vi "日志报警状态存储 (子VI).vi"() -> ()   [LabVIEW 2016, in "斯坦道CODMn.lvlib"]
uses:
  <vilib>/ptbypt/NI_PtbyPt.lvlib
panel:
  out "多列列表框":i32(listbox)
  out "CODMn工作状态":T1(ring)
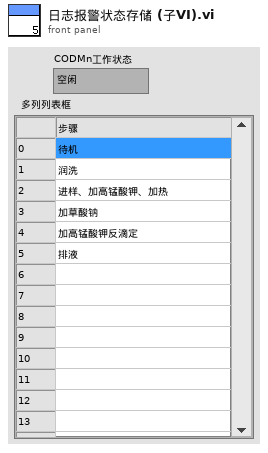
[diagram p1: front panel]
types:
  T1 = enum16{"空闲", "水样测试", "标样核查", "零点核查", "跨度核查", "空白测试", "平行样测试", "质控样", "空白校准", "标样校准", "加标回收"}
  T2 = cluster{"时间标识":timestamp, "设备":string, "日志信息":string, "备注":string}
  T3 = cluster{"时间标识":timestamp, "参数":string, "日志信息":string, "流程参数":string}
  T4 = cluster{"ORP故障":bool, "温控器故障":bool, "加热故障":bool, "高锰酸钾报警":bool, "草酸钠报警":bool, "测量错误":bool, "校零错误":bool, "校标错误":bool, " 进水样超量程":bool, "排液阀故障":bool, "60分钟超时报警":bool, "进样无液体报警":bool}
  T5 = cluster{"时间标识":timestamp, "设备":string, "日志信息":string, "流程参数":string}
  T6 = cluster{"测量量程":dbl, "测量精度":dbl, "测量间隔":dbl, "消解温度":dbl, "消解时长":dbl, "空白校准时间":timestamp, "曲线截距":dbl, "曲线斜率":dbl, "测量检出限":dbl, "测量信号值":dbl, "线性相关系数":dbl, "二次多项式系数":dbl, "标样校准时间":timestamp, "稀释倍数":dbl, "三项式系数":dbl, "空白标定系数":dbl, "量程系数":dbl, "F0/ORPA":dbl, "F1/ORPB":dbl, "F2/ORPK":dbl, "F3":dbl, "F4":dbl, "F5":dbl, "F6":dbl, "F7":dbl, "X0/滴定数":dbl, "量程":dbl}
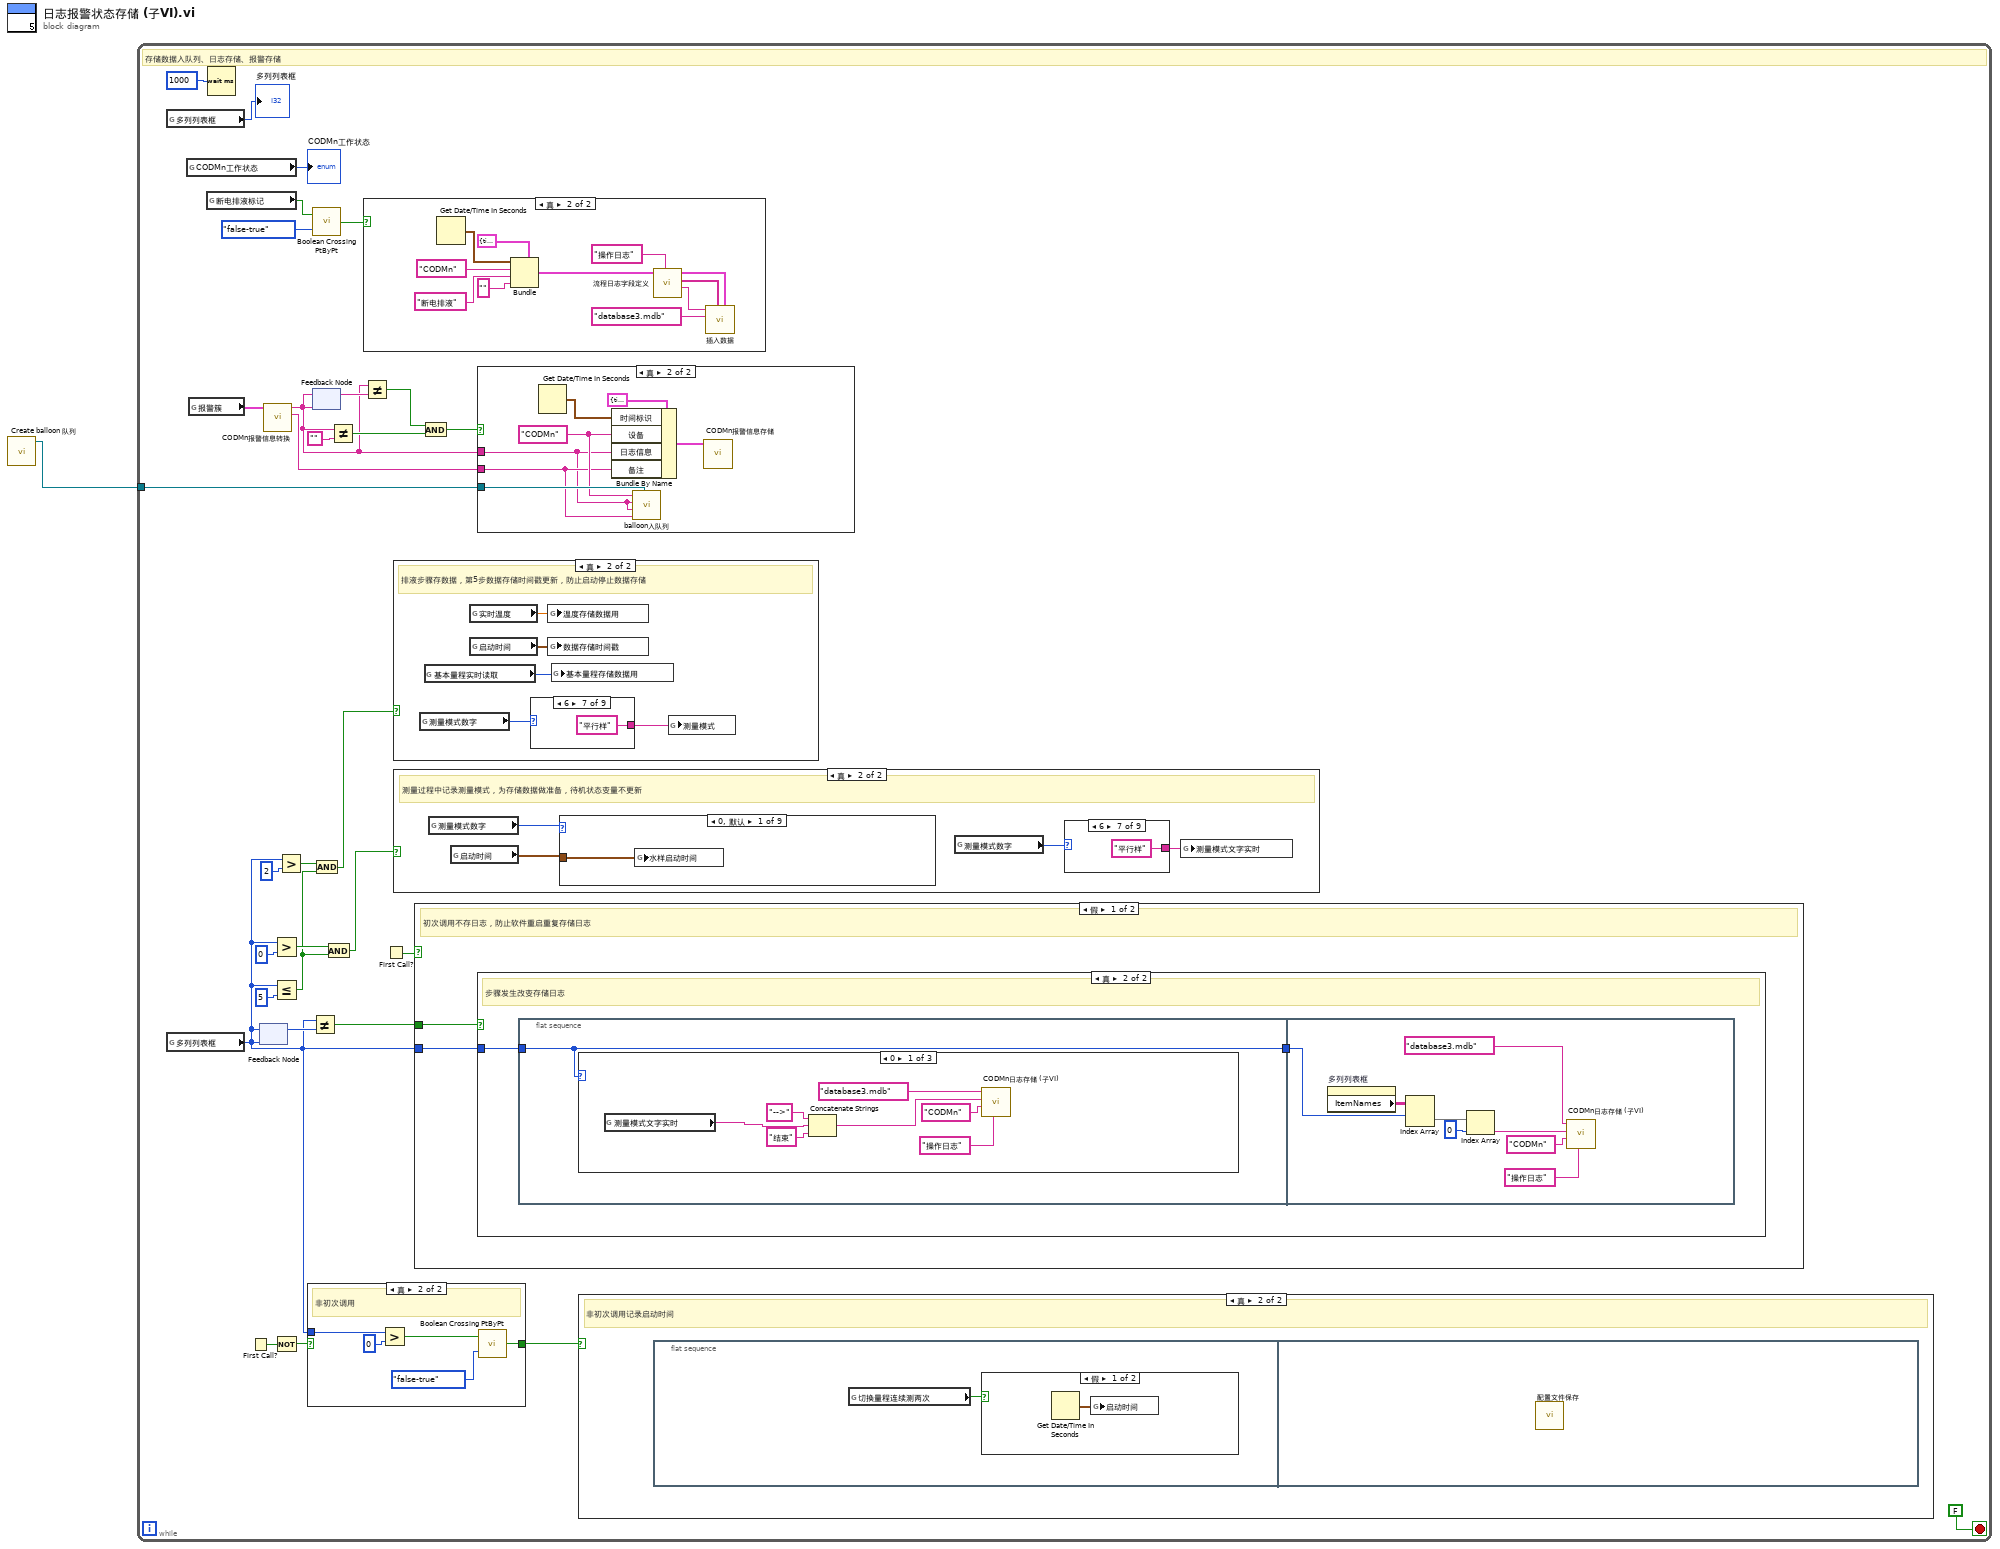
[diagram p0: block diagram]
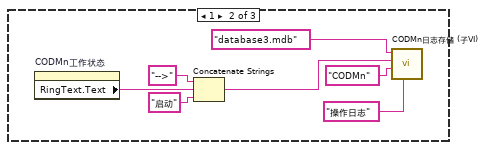
[diagram p3: hidden frame]
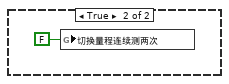
[diagram p10: hidden frame]
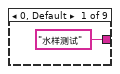
[diagram p12: hidden frame]
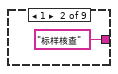
[diagram p13: hidden frame]
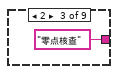
[diagram p14: hidden frame]
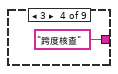
[diagram p15: hidden frame]
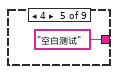
[diagram p16: hidden frame]
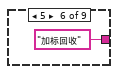
[diagram p17: hidden frame]
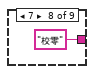
[diagram p18: hidden frame]
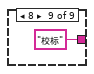
[diagram p19: hidden frame]
diagram:
  n1 = call "Create balloon 队列.vi"() -> ("队列输出"=w1:refnum<queue>)  [unwired: 11 in]
  n2 = while {
    tunnel: w1 -> [w2]
    stop <- FALSE stop-if-true
    # "存储数据入队列、日志存储、报警存储"
    n3 = global read "运行时序全局变量.vi" "多列列表框"() -> (→"多列列表框":i32)
    n4 = global read "运行时序全局变量.vi" "多列列表框"() -> (w6:i32)
    n5 = global read "COD测量模式全局.vi" "CODMn工作状态"() -> (→"CODMn工作状态":T1)
    n6 = global read "COD内部交互全局.vi" "报警簇"() -> (w13:T4)
    n7 = global read "COD内部交互全局.vi" "断电排液标记"() -> (w12:bool)
    n8 = Wait (ms)(milliseconds to wait=u32 1000 ("等待时间（毫秒）")) -> ()  [unwired: 1 out]
    n9 = First Call?() -> (First Call?: T/F=w16:bool)
    n10 = feedback #1(w6) -> (w27:i32)
    n11 = feedback-in #1(w6) -> ()
    n12 = call "CODMn报警信息转换.vi"("报警簇"=w13) -> ("CODMN报警信息备注"=w3:string, "CODMN报警信息"=w17:string)  [unwired: 9 in]
    n13 = Greater?(x=w6, y=u16 0) -> (0:w32:bool)
    n14 = Less Or Equal?(x=w6, y=u16 5) -> (x <= y?=w7:bool)
    n15 = Not(x=w16) -> (.not. x?=w14:bool)
    n16 = Greater?(x=w6, y=u16 2) -> (0:w8:bool)
    n17 = case shown="真" w14 {
      selector: w14 -> [w60 _]
      tunnel: w6 -> [_ w62]
      tunnel: [w60 w61] -> w15
      frame False {
      }
      frame True {
        # "非初次调用"
        n18 = Greater?(x=w62, y=u16 0) -> (0:w65:bool)
        n19 = call <vilib>:"Boolean Crossing PtByPt.vi"("direction"=enum16{"either", "false-true", "true-false"}."false-true", "input"=w65) -> ("crossing"=w61:bool)  [unwired: 1 in]
      }
    }
    n20 = Not Equal?(x=w6, y=w27) -> (x != y?=w28:bool)
    n21 = call <vilib>:"Boolean Crossing PtByPt.vi"("direction"=enum16{"either", "false-true", "true-false"}."false-true", "input"=w12) -> ("crossing"=w23:bool)  [unwired: 1 in]
    n22 = feedback #2(w17) -> (w18:string)
    n23 = feedback-in #2(w17) -> ()
    n24 = And(x=w8, y=w7) -> (x .and. y?=w5:bool)
    n25 = And(x=w32, y=w7) -> (x .and. y?=w4:bool)
    n26 = Not Equal?(x=w17, y="") -> (x != y?=w22:bool)
    n27 = Not Equal?(x=w17, y=w18) -> (x != y?=w19:bool)
    n28 = case shown="真" w23 {
      frame False {
      }
      frame True {
        n29 = Get Date/Time In Seconds() -> (seconds since 1Jan1904=w78:timestamp)
        n30 = Bundle(cluster=T3 {"时间标识"=timestamp(0 s since 1904-01-01), "参数"="", "日志信息"="", "流程参数"=""} ("data in"), "时间标识"=w78, "参数"="CODMn" ("table输入"), "日志信息"="断电排液", "流程参数"="" ("table输入")) -> (w76:T3)
        n31 = call "流程日志字段定义.vi"("table输入"="操作日志", "data in"=w76) -> ("table输出"=w81:string, "columns"=w82:string[], "data out"=w83:T5)  [unwired: 7 in]
        n32 = call "插入数据.vi"("data"=w83, "columns"=w82, "database"="database3.mdb", "table"=w81) -> ()  [unwired: 7 in, 1 out]
      }
    }
    n33 = First Call?() -> (First Call?: T/F=w29:bool)
    n34 = case shown="真" w5 {
      frame False {
      }
      frame True {
        # "排液步骤存数据，第5步数据存储时间戳更新，防止启动停止数据存储"
        n35 = global read "COD内部交互全局.vi" "测量模式数字"() -> (w108:i32)
        n36 = global read "COD内部交互全局.vi" "基本量程实时读取"() -> (w110:enum16{"L", "H", "AUTO"})
        n37 = global read "COD内部交互全局.vi" "实时温度"() -> (w111:dbl)
        n38 = global read "CODMn断电保存全局变量.vi" "启动时间"() -> (w112:timestamp)
        n39 = case shown="6" w108 {
          tunnel: ["水样测试" ("测量模式") "标样核查" ("测量模式") "零点核查" ("测量模式") "跨度核查" ("测量模式") "空白测试" ("测量模式") "加标回收" ("测量模式") "平行样" ("测量模式") "校零" ("测量模式") "校标" ("测量模式")] -> w109
          frame 0, Default {
          }
          frame 1 {
          }
          frame 2 {
          }
          frame 3 {
          }
          frame 4 {
          }
          frame 5 {
          }
          frame 6 {
          }
          frame 7 {
          }
          frame 8 {
          }
        }
        n40 = global write "COD内部交互全局.vi" "温度存储数据用"(w111) -> ()
        n41 = global write "COD内部交互全局.vi" "数据存储时间戳"(w112) -> ()
        n42 = global write "COD内部交互全局.vi" "基本量程存储数据用"(w110) -> ()
        n43 = global write "COD测量模式全局.vi" "测量模式"(w109) -> ()
      }
    }
    n44 = case shown="真" w4 {
      frame False {
      }
      frame True {
        # "测量过程中记录测量模式，为存储数据做准备，待机状态变量不更新"
        n45 = global read "COD内部交互全局.vi" "测量模式数字"() -> (w89:i32)
        n46 = global read "CODMn断电保存全局变量.vi" "启动时间"() -> (w90:timestamp)
        n47 = case shown="0, 默认" w89 {
          tunnel: w90 -> [w100 _ _ _ _ w101 _ w102 w105]
          frame 0, Default {
            n48 = global write "COD测量模式全局.vi" "水样启动时间"(w100) -> ()
          }
          frame 1 {
          }
          frame 2 {
          }
          frame 3 {
          }
          frame 4 {
          }
          frame 5 {
            n49 = global write "COD测量模式全局.vi" "加标回收启动时间"(w101) -> ()
          }
          frame 6 {
          }
          frame 7 {
            n50 = global read "CODMn断电保存全局变量.vi" "CODMn仪器参数"() -> (w104:T6)
            n51 = Bundle By Name(cluster=w104, "空白校准时间"=w102) -> (w103:T6)
            n52 = global write "CODMn断电保存全局变量.vi" "CODMn仪器参数"(w103) -> ()
          }
          frame 8 {
            n53 = global read "CODMn断电保存全局变量.vi" "CODMn仪器参数"() -> (w107:T6)
            n54 = Bundle By Name(cluster=w107, "标样校准时间"=w105) -> (w106:T6)
            n55 = global write "CODMn断电保存全局变量.vi" "CODMn仪器参数"(w106) -> ()
          }
        }
        n56 = global read "COD内部交互全局.vi" "测量模式数字"() -> (w87:i32)
        n57 = case shown="6" w87 {
          tunnel: ["水样测试" ("测量模式") "标样核查" ("测量模式") "零点核查" ("测量模式") "跨度核查" ("测量模式") "空白测试" ("测量模式") "加标回收" ("测量模式") "平行样" ("测量模式") "校零" ("测量模式") "校标" ("测量模式")] -> w88
          frame 0, Default {
          }
          frame 1 {
          }
          frame 2 {
          }
          frame 3 {
          }
          frame 4 {
          }
          frame 5 {
          }
          frame 6 {
          }
          frame 7 {
          }
          frame 8 {
          }
        }
        n58 = global write "COD测量模式全局.vi" "测量模式文字实时"(w88) -> ()
      }
    }
    n59 = case shown="假" w29 {
      tunnel: w28 -> [w34 _]
      tunnel: w6 -> [w33 _]
      frame False {
        # "初次调用不存日志，防止软件重启重复存储日志"
        n60 = case shown="真" w34 {
          tunnel: w33 -> [_ w36]
          frame False {
          }
          frame True {
            # "步骤发生改变存储日志"
            n61 = flat-sequence {
              tunnel: w36 -> [w37]
              tunnel: [w37] -> w35
              tunnel: w35 -> [w57]
              frame #0 {
                n62 = case shown="0" w37 {
                  frame 0 {
                    n63 = global read "COD测量模式全局.vi" "测量模式文字实时"() -> (w38:string)
                    n64 = Concatenate Strings("-->", w38, "结束" ("字符串")) -> (w44:string)
                    n65 = call "CODMn日志存储 (子VI).vi"("table输入"="操作日志", "参数"="CODMn" ("table输入"), "日志信息"=w44, "database"="database3.mdb") -> ()  [unwired: 8 in]
                  }
                  frame 1 {
                    n66 = property on="CODMn工作状态" class="Enum (严格)"() -> ("RingText.Text"=w45:string)  [unwired: 2 in, 2 out]
                    n67 = Concatenate Strings("-->", w45, "启动" ("字符串")) -> (w46:string)
                    n68 = call "CODMn日志存储 (子VI).vi"("table输入"="操作日志", "参数"="CODMn" ("table输入"), "日志信息"=w46, "database"="database3.mdb") -> ()  [unwired: 8 in]
                  }
                  frame 2, Default {
                  }
                }
              }
              frame #1 {
                n69 = property on="多列列表框" class="MCListbox (严格)"() -> ("ItemNames"=w52:string[][])  [unwired: 2 in, 2 out]
                n70 = Index Array(array=w52, index (row)=w57) -> (element=w55:string[])  [unwired: 1 in]
                n71 = Index Array(array=w55, index=0 ("索引")) -> (element=w53:string)
                n72 = call "CODMn日志存储 (子VI).vi"("table输入"="操作日志", "参数"="CODMn" ("table输入"), "日志信息"=w53, "database"="database3.mdb") -> ()  [unwired: 8 in]
              }
            }
          }
        }
      }
      frame True {
      }
    }
    n73 = And(x=w19, y=w22) -> (x .and. y?=w20:bool)
    n74 = case shown="真" w20 {
      tunnel: w17 -> [_ w66]
      tunnel: w3 -> [_ w67]
      tunnel: w2 -> [_ w69]
      frame False {
      }
      frame True {
        w68 = "CODMn" ("设备")
        n75 = Get Date/Time In Seconds() -> (seconds since 1Jan1904=w72:timestamp)
        n76 = Bundle By Name(cluster=T2 {"时间标识"=timestamp(0 s since 1904-01-01), "设备"="", "日志信息"="", "备注"=""} ("data in"), "时间标识"=w72, "设备"=w68, "日志信息"=w66, "备注"=w67) -> (w70:T2)
        n77 = call "balloon入队列.vi"("队列"=w69, "故障详情"=w67, "告警信息"=w66, "故障信息"=w66, "参数名称"=w68) -> ()  [unwired: 6 in, 1 out]
        n78 = call "CODMn报警信息存储.vi"("data in"=w70) -> ()  [unwired: 10 in, 1 out]
      }
    }
    n79 = case shown="真" w15 {
      frame False {
      }
      frame True {
        # "非初次调用记录启动时间"
        n80 = flat-sequence {
          frame #0 {
            n81 = global read "COD内部交互全局.vi" "切换量程连续测两次"() -> (w84:bool)
            n82 = case shown="假" w84 {
              frame False {
                n83 = Get Date/Time In Seconds() -> (seconds since 1Jan1904=w85:timestamp)
                n84 = global write "CODMn断电保存全局变量.vi" "启动时间"(w85) -> ()
              }
              frame True {
                n85 = global write "COD内部交互全局.vi" "切换量程连续测两次"(FALSE ("切换量程连续测两次")) -> ()
              }
            }
          }
          frame #1 {
            n86 = call "配置文件保存.vi"() -> ()  [unwired: 12 in]
          }
        }
      }
    }
  }
